vi "DisableControls.vi"(7 "Enable (T)":bool, 8 "error in (no error)":errorcluster, 10 "Device Properties In":T1={"Configuration Mode"=enum."Constant Power (AC)", "Phases"=[{"Handle"="", "Name"="", "Phase Select"=1, "Instrument Options"="", "id query (T)"=TRUE, "reset device (T)"=TRUE, "Load Short Circuited"=FALSE, "Line Synchronization"=FALSE, "Load Current (A/Arms)"=1.0, "Load Voltage (V/Vrms)"=0.0, "Load Power (W)"=0.0, "Load Resistance (Ohms)"=0.0, "Load Current Peak Limit (A)"=0.0, "Load Current Limit (A/Arms)"=0.0, "Load Power Limit (W)"=0.0, "Synch Frequency (Hz)"=0.0, "Priority"=enum."CF Only", "Crest Factor"=0.0, "Power Factor"=0.0, "Slew Rate"={"Rise Slew Rate (A/ms)"=0, "Fall Slew Rate (A/ms)"=0}, "LC/RLC Mode"={"Capacitance (uF)"=0, "Inductance (uH)"=0, "Series Resistance (Ohm)"=0.0, "Parallel Resistance (Ohm)"=0.0}, "Timing"={"TimingOn"=enum."", "Hours"=0, "Minutes"=0, "Seconds"=0.0, "CutoffVoltage"=0.0}, "Connected"=FALSE}]} {"Phases"."Phase Select" items=["Phase ALL", "Phase A", "Phase B", "Phase C"]}, 11 "Cluster":refnum<vi>) -> (0 "Error Out":errorcluster, 2 "Device Properties Out":T1={"Configuration Mode"=enum."Constant Power (AC)", "Phases"=[{"Handle"="", "Name"="", "Phase Select"=1, "Instrument Options"="", "id query (T)"=TRUE, "reset device (T)"=TRUE, "Load Short Circuited"=FALSE, "Line Synchronization"=FALSE, "Load Current (A/Arms)"=1.0, "Load Voltage (V/Vrms)"=0.0, "Load Power (W)"=0.0, "Load Resistance (Ohms)"=0.0, "Load Current Peak Limit (A)"=0.0, "Load Current Limit (A/Arms)"=0.0, "Load Power Limit (W)"=0.0, "Synch Frequency (Hz)"=0.0, "Priority"=enum."CF Only", "Crest Factor"=0.0, "Power Factor"=0.0, "Slew Rate"={"Rise Slew Rate (A/ms)"=0, "Fall Slew Rate (A/ms)"=0}, "LC/RLC Mode"={"Capacitance (uF)"=0, "Inductance (uH)"=0, "Series Resistance (Ohm)"=0.0, "Parallel Resistance (Ohm)"=0.0}, "Timing"={"TimingOn"=enum."", "Hours"=0, "Minutes"=0, "Seconds"=0.0, "CutoffVoltage"=0.0}, "Connected"=FALSE}]} {"Phases"."Phase Select" items=["Phase ALL", "Phase A", "Phase B", "Phase C"]})   [LabVIEW 2018, in "AcPwrPlugins.lvlib" / "ChromaAcLoad.lvclass"]
doc: "This VI disables the controls in the phases cluster based on the Configuration Mode control. This will enable the user to only change the values of the controls that are allowed by that mode."
uses:
  ChromaAcLoad.lvclass
  TypeDefs/DeviceProperties.ctl
panel:
  # "1"
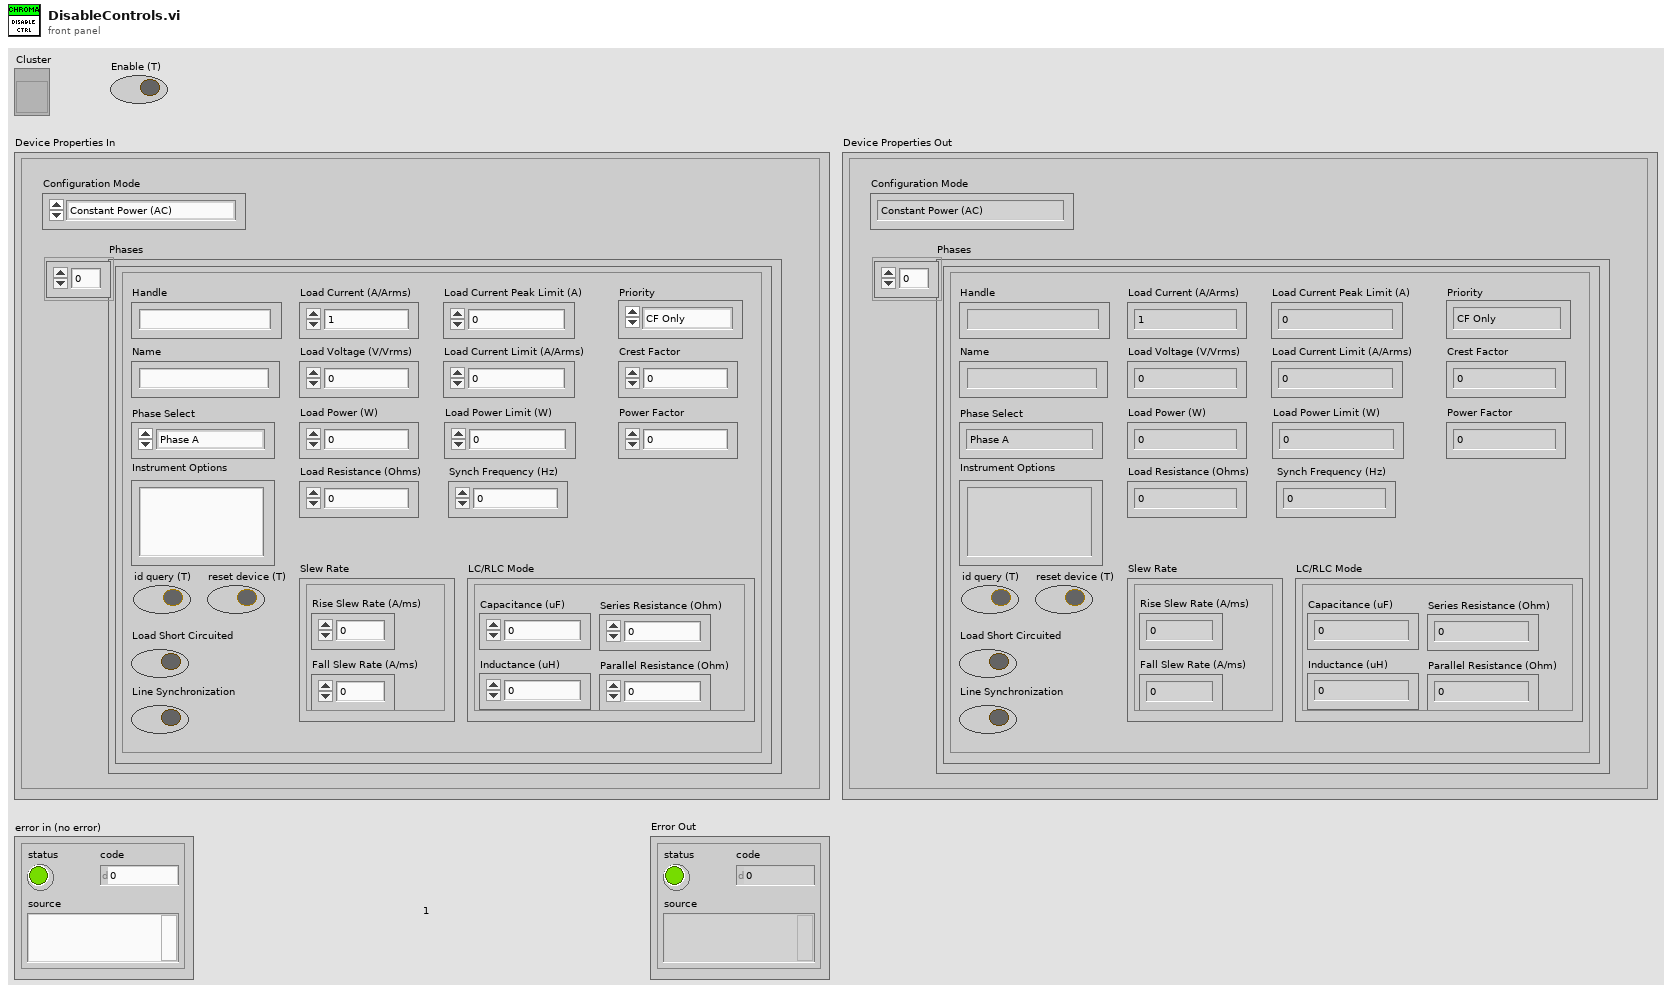
[diagram p1: front panel]
types:
  T1 = typedef "AcPwrPlugins.lvlib/ChromaAcLoad.lvclass/DeviceProperties.ctl" = cluster{"Configuration Mode":enum16{"Constant Voltage (DC)", "Constant Power (DC)", "Constant Power (AC)", "Constant Current (DC)", "Constant Current (AC)", "Constant Resistance (DC)", "Constant Resistance (AC)", "Rectified Mode (DC)", "Inrush (AC)", "RLC CP (AC)", "RLC (AC)"}, "Phases":cluster{"Handle":string, "Name":string, "Phase Select":i32, "Instrument Options":string, "id query (T)":bool, "reset device (T)":bool, "Load Short Circuited":bool, "Line Synchronization":bool, "Load Current (A/Arms)":dbl, "Load Voltage (V/Vrms)":dbl, "Load Power (W)":dbl, "Load Resistance (Ohms)":dbl, "Load Current Peak Limit (A)":dbl, "Load Current Limit (A/Arms)":dbl, "Load Power Limit (W)":dbl, "Synch Frequency (Hz)":dbl, "Priority":enum16{"CF Only", "PF Only", "Both (CF)", "Both (PF)"}, "Crest Factor":dbl, "Power Factor":dbl, "Slew Rate":cluster{"Rise Slew Rate (A/ms)":i32, "Fall Slew Rate (A/ms)":i32}, "LC/RLC Mode":cluster{"Capacitance (uF)":i32, "Inductance (uH)":i32, "Series Resistance (Ohm)":dbl, "Parallel Resistance (Ohm)":dbl}, "Timing":cluster{"TimingOn":enum16{""}, "Hours":u32, "Minutes":u32, "Seconds":dbl, "CutoffVoltage":dbl}, "Connected":bool}[]}
  T2 = enum8{"Enabled", "Disabled", "Disabled and Grayed Out"}
  T3 = enum16{"Constant Voltage (DC)", "Constant Power (DC)", "Constant Power (AC)", "Constant Current (DC)", "Constant Current (AC)", "Constant Resistance (DC)", "Constant Resistance (AC)", "Rectified Mode (DC)", "Inrush (AC)", "RLC CP (AC)", "RLC (AC)"}
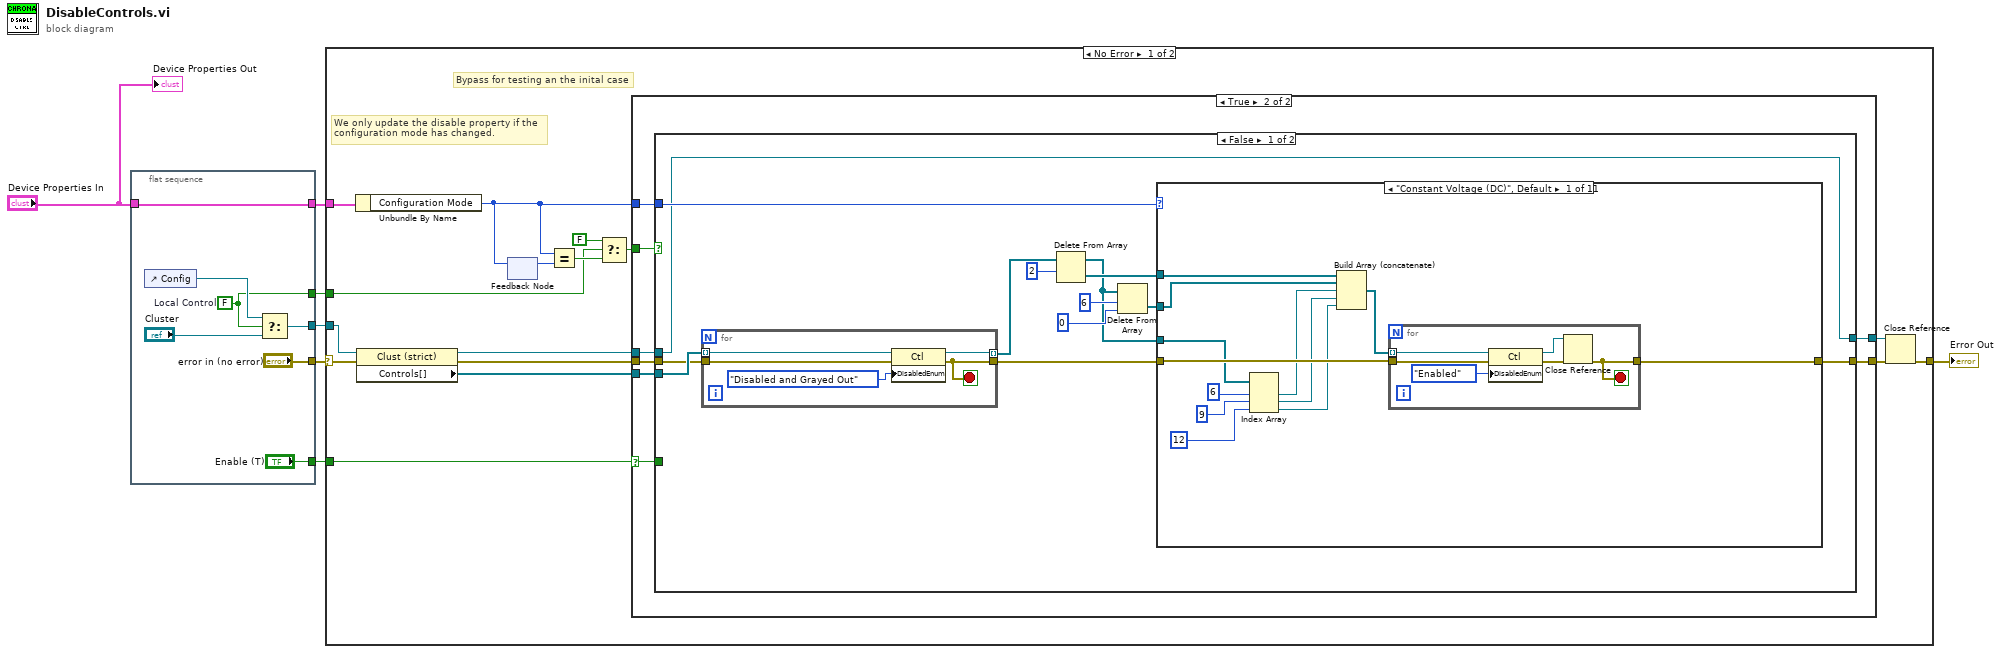
[diagram p0: block diagram]
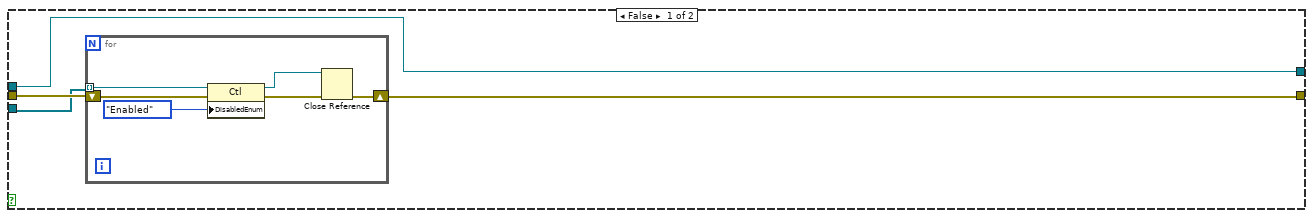
[diagram p2: hidden frame]
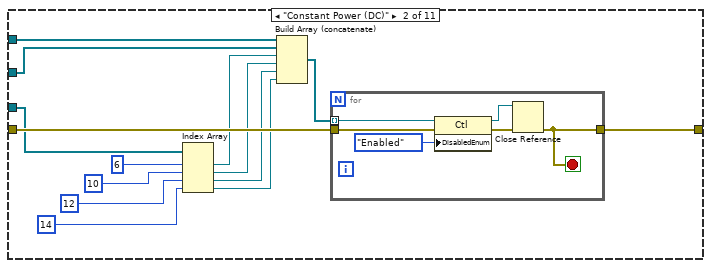
[diagram p3: hidden frame]
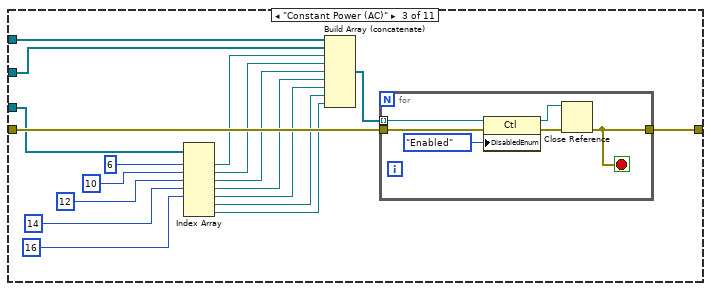
[diagram p4: hidden frame]
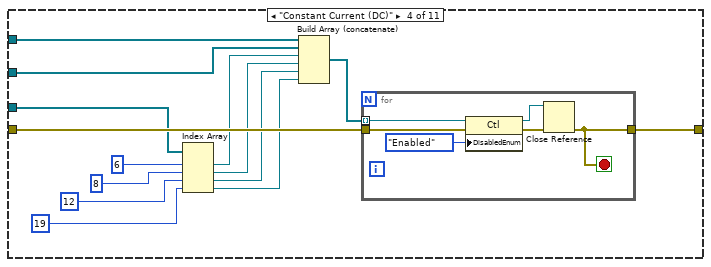
[diagram p5: hidden frame]
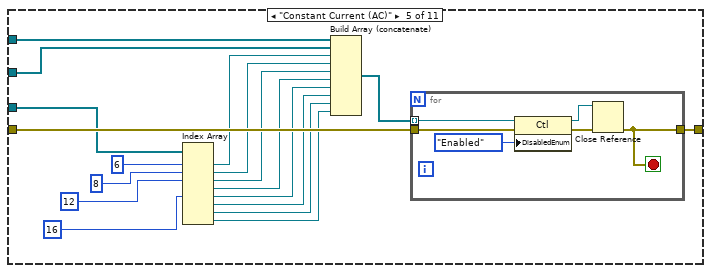
[diagram p6: hidden frame]
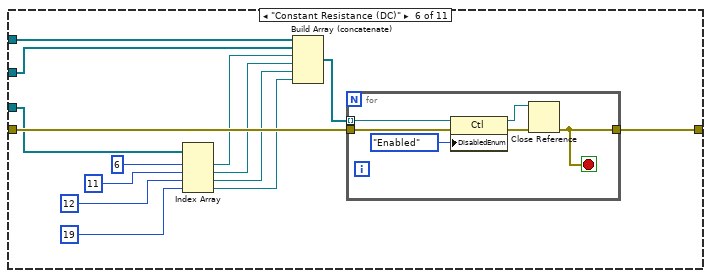
[diagram p7: hidden frame]
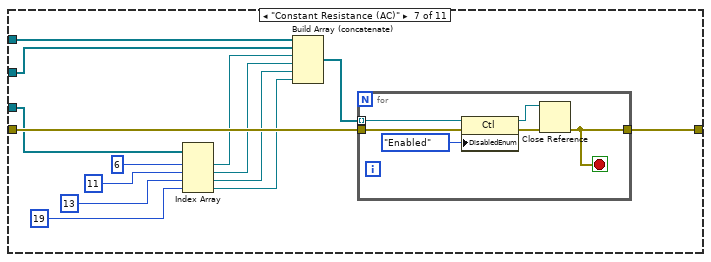
[diagram p8: hidden frame]
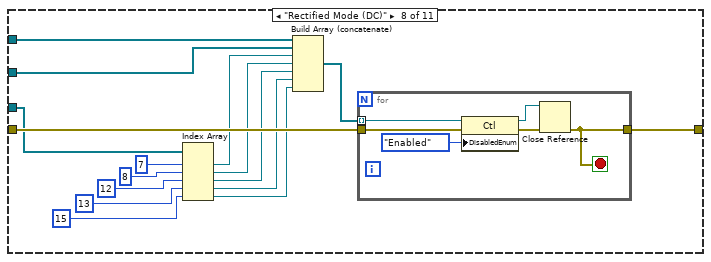
[diagram p9: hidden frame]
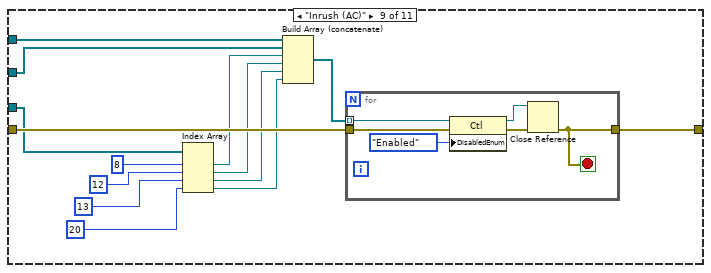
[diagram p10: hidden frame]
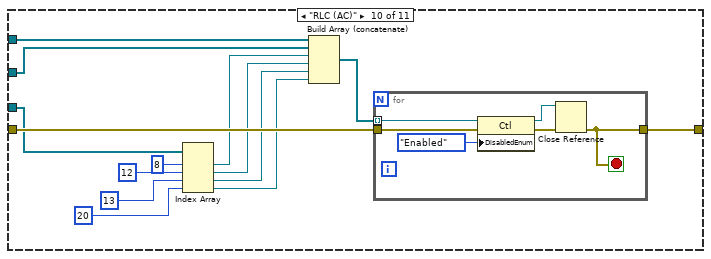
[diagram p11: hidden frame]
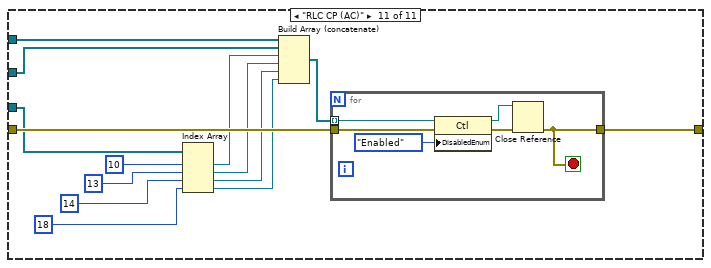
[diagram p12: hidden frame]
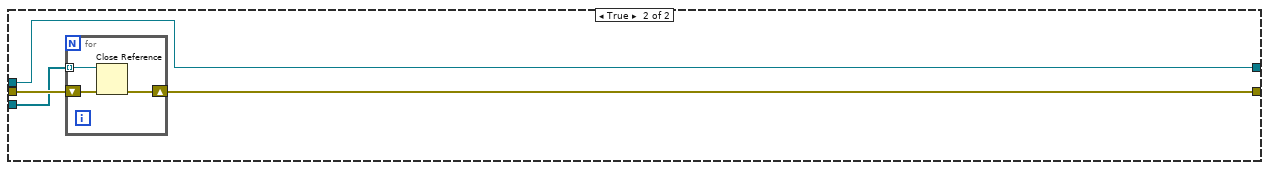
[diagram p13: hidden frame]
diagram:
  n1 = flat-sequence {
    tunnel: ["error in (no error)"] -> w6
    tunnel: [w13] -> w5
    tunnel: [w9] -> w4
    tunnel: ["Enable (T)"] -> w3
    tunnel: "Device Properties In" -> [w10]
    tunnel: [w10] -> w1
    frame #0 {
      w9 = FALSE  # Local Control
      n2 = control-ref of="Config"() -> (w11:refnum<vi>)
      n3 = Select(t=w11, s=w9, f="Cluster") -> (s? t:f=w13:refnum<vi>)
    }
  }
  n4 = case shown="No Error" w6 {
    selector: w6 -> [w24 w302]
    tunnel: [w23 w302] -> w7
    tunnel: w5 -> [w26 _]
    tunnel: w4 -> [w16 _]
    tunnel: w3 -> [w18 _]
    tunnel: w1 -> [w17 _]
    frame No Error {
      # "Bypass for testing an the inital case"
      # "We only update the disable property if the\nconfiguration mode has changed."
      n5 = Unbundle By Name(w17) -> ("Configuration Mode"=w25:T3)
      n6 = property class="Clust (strict)"(reference=w26, error in=w24) -> (reference out=w28:refnum<vi>, error out=w29:errorcluster, "Controls[]"=w27:refnum<vi>[])
      n7 = feedback #1() -> (w15:T3)  [unwired: 1 in]
      n8 = feedback-in #1(w25) -> ()
      n9 = Equal?(x=w25, y=w15) -> (x = y?=w21:bool)
      n10 = Select(t=FALSE, s=w16, f=w21) -> (s? t:f=w20:bool)
      n11 = case shown="True" w18 {
        selector: w18 -> [_ w47]
        tunnel: [w32 w48] -> w30
        tunnel: w29 -> [w34 w46]
        tunnel: w28 -> [w31 w45]
        tunnel: w27 -> [w33 w44]
        tunnel: w25 -> [_ w43]
        tunnel: w20 -> [_ w42]
        tunnel: [w31 w41] -> w22
        frame False {
          n12 = for {
            shift-right: [w36] -> w32
            shift-left: w34 -> [w39]
            tunnel: w33 -> [w38] mode=indexing
            n13 = property on="Property Node" class="Ctl"(reference=w38, error in=w39, "DisabledEnum"=T2."Enabled" ("Disabled")) -> (reference out=w35:refnum<vi>, error out=w37:errorcluster)
            n14 = Close Reference(reference=w35, error in (no error)=w37) -> (error out=w36:errorcluster)
          }
        }
        frame True {
          n15 = case shown="False" w42 {
            tunnel: [w61 w296] -> w48
            tunnel: w46 -> [w49 w298]
            tunnel: w45 -> [w52 w295]
            tunnel: w44 -> [w51 w297]
            tunnel: w43 -> [w59 _]
            tunnel: [w52 w295] -> w41
            tunnel: w47 -> [_ _]
            frame False {
              n16 = for {
                tunnel: [w65] -> w50 mode=indexing
                tunnel: w51 -> [w64] mode=indexing
                tunnel: w49 -> [w63]
                tunnel: [w62] -> w60
                stop <- w62 stop-if-true
                n17 = property class="Ctl"(reference=w64, error in=w63, "DisabledEnum"=T2."Disabled and Grayed Out" ("Disabled")) -> (reference out=w65:refnum<vi>, error out=w62:errorcluster)
              }
              n18 = Delete From Array(array=w50, length=2) -> (deleted portion=w55:refnum<vi>[], array with subset deleted=w53:refnum<vi>[])  [unwired: 1 in]
              n19 = Delete From Array(array=w53, length=6, index=0) -> (deleted portion=w54:refnum<vi>[])  [unwired: 1 out]
              n20 = case shown="\"Constant Voltage (DC)\", Default" w59 {
                tunnel: [w77 w97 w121 w141 w165 w185 w205 w227 w247 w267 w287] -> w61
                tunnel: w60 -> [w78 w98 w122 w142 w166 w186 w206 w228 w248 w268 w288]
                tunnel: w55 -> [w69 w89 w109 w131 w153 w175 w195 w217 w242 w260 w279]
                tunnel: w54 -> [w68 w88 w108 w130 w152 w174 w194 w216 w241 w259 w278]
                tunnel: w53 -> [w67 w87 w107 w129 w151 w173 w193 w215 w240 w258 w277]
                frame "Constant Voltage (DC)", Default {
                  n21 = Index Array(array=w67, index #1=6 ("index"), index #2=9 ("index"), index #3=12 ("index")) -> (element #1=w74:refnum<vi>, element #2=w73:refnum<vi>, element #3=w71:refnum<vi>)
                  n22 = Build Array (concatenate)(w69, w68, w74, w73, w71) -> (w76:refnum<vi>[])
                  n23 = for {
                    tunnel: w78 -> [w84]
                    tunnel: [w79] -> w77
                    tunnel: w76 -> [w82] mode=indexing
                    stop <- w79 stop-if-true
                    n24 = property class="Ctl"(reference=w82, error in=w84, "DisabledEnum"=T2."Enabled" ("Disabled")) -> (reference out=w80:refnum<vi>, error out=w81:errorcluster)
                    n25 = Close Reference(reference=w80, error in (no error)=w81) -> (error out=w79:errorcluster)
                  }
                }
                frame "Constant Power (DC)" {
                  n26 = Index Array(array=w87, index #1=6 ("index"), index #2=10 ("index"), index #3=12 ("index"), index #4=14 ("index")) -> (element #1=w94:refnum<vi>, element #2=w93:refnum<vi>, element #3=w90:refnum<vi>, element #4=w86:refnum<vi>)
                  n27 = Build Array (concatenate)(w89, w88, w94, w93, w90, w86) -> (w96:refnum<vi>[])
                  n28 = for {
                    tunnel: w98 -> [w104]
                    tunnel: [w99] -> w97
                    tunnel: w96 -> [w102] mode=indexing
                    stop <- w99 stop-if-true
                    n29 = property class="Ctl"(reference=w102, error in=w104, "DisabledEnum"=T2."Enabled" ("Disabled")) -> (reference out=w100:refnum<vi>, error out=w101:errorcluster)
                    n30 = Close Reference(reference=w100, error in (no error)=w101) -> (error out=w99:errorcluster)
                  }
                }
                frame "Constant Power (AC)" {
                  n31 = Index Array(array=w107, index #1=6 ("index"), index #2=10 ("index"), index #3=12 ("index"), index #4=14 ("index"), index #5=16 ("index")) -> (element #1=w118:refnum<vi>, element #2=w117:refnum<vi>, element #3=w115:refnum<vi>, element #4=w112:refnum<vi>, element #5=w111:refnum<vi>, element #6=w110:refnum<vi>, element #7=w105:refnum<vi>)  [unwired: 2 in]
                  n32 = Build Array (concatenate)(w109, w108, w118, w117, w115, w112, w111, w110, w105) -> (w120:refnum<vi>[])
                  n33 = for {
                    tunnel: w122 -> [w128]
                    tunnel: [w123] -> w121
                    tunnel: w120 -> [w126] mode=indexing
                    stop <- w123 stop-if-true
                    n34 = property class="Ctl"(reference=w126, error in=w128, "DisabledEnum"=T2."Enabled" ("Disabled")) -> (reference out=w124:refnum<vi>, error out=w125:errorcluster)
                    n35 = Close Reference(reference=w124, error in (no error)=w125) -> (error out=w123:errorcluster)
                  }
                }
                frame "Constant Current (DC)" {
                  n36 = Index Array(array=w129, index #1=6 ("index"), index #2=8 ("index"), index #3=12 ("index"), index #4=19 ("index")) -> (element #1=w138:refnum<vi>, element #2=w137:refnum<vi>, element #3=w135:refnum<vi>, element #4=w132:refnum<vi>)
                  n37 = Build Array (concatenate)(w131, w130, w138, w137, w135, w132) -> (w140:refnum<vi>[])
                  n38 = for {
                    tunnel: w142 -> [w148]
                    tunnel: [w143] -> w141
                    tunnel: w140 -> [w146] mode=indexing
                    stop <- w143 stop-if-true
                    n39 = property class="Ctl"(reference=w146, error in=w148, "DisabledEnum"=T2."Enabled" ("Disabled")) -> (reference out=w144:refnum<vi>, error out=w145:errorcluster)
                    n40 = Close Reference(reference=w144, error in (no error)=w145) -> (error out=w143:errorcluster)
                  }
                }
                frame "Constant Current (AC)" {
                  n41 = Index Array(array=w151, index #1=6 ("index"), index #2=8 ("index"), index #3=12 ("index"), index #5=16 ("index")) -> (element #1=w162:refnum<vi>, element #2=w161:refnum<vi>, element #3=w159:refnum<vi>, element #4=w157:refnum<vi>, element #5=w156:refnum<vi>, element #6=w155:refnum<vi>, element #7=w154:refnum<vi>, element #8=w150:refnum<vi>)  [unwired: 4 in]
                  n42 = Build Array (concatenate)(w153, w152, w162, w161, w159, w157, w156, w155, w154, w150) -> (w164:refnum<vi>[])
                  n43 = for {
                    tunnel: w166 -> [w172]
                    tunnel: [w167] -> w165
                    tunnel: w164 -> [w170] mode=indexing
                    stop <- w167 stop-if-true
                    n44 = property class="Ctl"(reference=w170, error in=w172, "DisabledEnum"=T2."Enabled" ("Disabled")) -> (reference out=w168:refnum<vi>, error out=w169:errorcluster)
                    n45 = Close Reference(reference=w168, error in (no error)=w169) -> (error out=w167:errorcluster)
                  }
                }
                frame "Constant Resistance (DC)" {
                  n46 = Index Array(array=w173, index #1=6 ("index"), index #2=11 ("index"), index #3=12 ("index"), index #4=19 ("index")) -> (element #1=w182:refnum<vi>, element #2=w181:refnum<vi>, element #3=w178:refnum<vi>, element #4=w176:refnum<vi>)
                  n47 = Build Array (concatenate)(w175, w174, w182, w181, w178, w176) -> (w184:refnum<vi>[])
                  n48 = for {
                    tunnel: w186 -> [w192]
                    tunnel: [w187] -> w185
                    tunnel: w184 -> [w190] mode=indexing
                    stop <- w187 stop-if-true
                    n49 = property class="Ctl"(reference=w190, error in=w192, "DisabledEnum"=T2."Enabled" ("Disabled")) -> (reference out=w188:refnum<vi>, error out=w189:errorcluster)
                    n50 = Close Reference(reference=w188, error in (no error)=w189) -> (error out=w187:errorcluster)
                  }
                }
                frame "Constant Resistance (AC)" {
                  n51 = Index Array(array=w193, index #1=6 ("index"), index #2=11 ("index"), index #3=13 ("index"), index #4=19 ("index")) -> (element #1=w202:refnum<vi>, element #2=w201:refnum<vi>, element #3=w198:refnum<vi>, element #4=w196:refnum<vi>)
                  n52 = Build Array (concatenate)(w195, w194, w202, w201, w198, w196) -> (w204:refnum<vi>[])
                  n53 = for {
                    tunnel: w206 -> [w212]
                    tunnel: [w207] -> w205
                    tunnel: w204 -> [w210] mode=indexing
                    stop <- w207 stop-if-true
                    n54 = property class="Ctl"(reference=w210, error in=w212, "DisabledEnum"=T2."Enabled" ("Disabled")) -> (reference out=w208:refnum<vi>, error out=w209:errorcluster)
                    n55 = Close Reference(reference=w208, error in (no error)=w209) -> (error out=w207:errorcluster)
                  }
                }
                frame "Rectified Mode (DC)" {
                  n56 = Index Array(array=w215, index #1=7 ("index"), index #2=8 ("index"), index #3=12 ("index"), index #4=13 ("index"), index #5=15 ("index")) -> (element #1=w224:refnum<vi>, element #2=w223:refnum<vi>, element #3=w220:refnum<vi>, element #4=w218:refnum<vi>, element #5=w214:refnum<vi>)
                  n57 = Build Array (concatenate)(w217, w216, w224, w223, w220, w218, w214) -> (w226:refnum<vi>[])
                  n58 = for {
                    tunnel: w228 -> [w234]
                    tunnel: [w229] -> w227
                    tunnel: w226 -> [w232] mode=indexing
                    stop <- w229 stop-if-true
                    n59 = property class="Ctl"(reference=w232, error in=w234, "DisabledEnum"=T2."Enabled" ("Disabled")) -> (reference out=w230:refnum<vi>, error out=w231:errorcluster)
                    n60 = Close Reference(reference=w230, error in (no error)=w231) -> (error out=w229:errorcluster)
                  }
                }
                frame "Inrush (AC)" {
                  n61 = Index Array(array=w240, index #1=8 ("index"), index #2=12 ("index"), index #3=13 ("index"), index #4=20 ("index")) -> (element #1=w245:refnum<vi>, element #2=w244:refnum<vi>, element #3=w243:refnum<vi>, element #4=w235:refnum<vi>)
                  n62 = Build Array (concatenate)(w242, w241, w245, w244, w243, w235) -> (w246:refnum<vi>[])
                  n63 = for {
                    tunnel: w248 -> [w254]
                    tunnel: [w249] -> w247
                    tunnel: w246 -> [w252] mode=indexing
                    stop <- w249 stop-if-true
                    n64 = property class="Ctl"(reference=w252, error in=w254, "DisabledEnum"=T2."Enabled" ("Disabled")) -> (reference out=w250:refnum<vi>, error out=w251:errorcluster)
                    n65 = Close Reference(reference=w250, error in (no error)=w251) -> (error out=w249:errorcluster)
                  }
                }
                frame "RLC (AC)" {
                  n66 = Index Array(array=w258, index #1=8 ("index"), index #2=12 ("index"), index #3=13 ("index"), index #4=20 ("index")) -> (element #1=w264:refnum<vi>, element #2=w263:refnum<vi>, element #3=w262:refnum<vi>, element #4=w261:refnum<vi>)
                  n67 = Build Array (concatenate)(w260, w259, w264, w263, w262, w261) -> (w266:refnum<vi>[])
                  n68 = for {
                    tunnel: w268 -> [w274]
                    tunnel: [w269] -> w267
                    tunnel: w266 -> [w272] mode=indexing
                    stop <- w269 stop-if-true
                    n69 = property class="Ctl"(reference=w272, error in=w274, "DisabledEnum"=T2."Enabled" ("Disabled")) -> (reference out=w270:refnum<vi>, error out=w271:errorcluster)
                    n70 = Close Reference(reference=w270, error in (no error)=w271) -> (error out=w269:errorcluster)
                  }
                }
                frame "RLC CP (AC)" {
                  n71 = Index Array(array=w277, index #1=10 ("index"), index #2=13 ("index"), index #3=14 ("index"), index #4=18 ("index")) -> (element #1=w284:refnum<vi>, element #2=w283:refnum<vi>, element #3=w280:refnum<vi>, element #4=w275:refnum<vi>)
                  n72 = Build Array (concatenate)(w279, w278, w284, w283, w280, w275) -> (w286:refnum<vi>[])
                  n73 = for {
                    tunnel: w288 -> [w294]
                    tunnel: [w289] -> w287
                    tunnel: w286 -> [w292] mode=indexing
                    stop <- w289 stop-if-true
                    n74 = property class="Ctl"(reference=w292, error in=w294, "DisabledEnum"=T2."Enabled" ("Disabled")) -> (reference out=w290:refnum<vi>, error out=w291:errorcluster)
                    n75 = Close Reference(reference=w290, error in (no error)=w291) -> (error out=w289:errorcluster)
                  }
                }
              }
            }
            frame True {
              n76 = for {
                shift-right: [w299] -> w296
                shift-left: w298 -> [w301]
                tunnel: w297 -> [w300] mode=indexing
                n77 = Close Reference(reference=w300, error in (no error)=w301) -> (error out=w299:errorcluster)
              }
            }
          }
        }
      }
      n78 = Close Reference(reference=w22, error in (no error)=w30) -> (error out=w23:errorcluster)
    }
    frame Error {
    }
  }
  "Error Out" <- w7
  "Device Properties Out" <- "Device Properties In"
